vi "OAXML_Load Configuration.vi"(8 "error in (not an error)":errorcluster, 11 "config file":path) -> (0 "error out":errorcluster, 1 "DAQ Configuration out":T1 {"pregain" format="%.2f"; "IEPE" items=["On", "Off", "None"]; "coupling" items=["DC", "AC"]; "engineering units" items=["custom..."=0, "V"=1, "A"=21, "C"=30, "pC"=31, "s"=32, "-"=29, "Pa"=2, "N"=20, "g"=3, "m/s^2"=4, "m/s"=5, "m"=6, "mm/s"=12, "mm"=13, "micron/s"=14, "micron"=15, "in/s^2"=7, "in/s"=8, "in"=9, "mil/s"=10, "mil"=11, "rad/s^2"=16, "rad/s"=17, "rad"=18, "deg/s^2"=26, "deg/s"=27, "deg"=28, "RPM"=22, "cycle/s^2"=23, "Hz"=24, "cycle"=25, "strain"=19]; "sensor sensitivity (mV/EU)" format="%.2f"; "dB reference" format="%.1e"}, 2 "param out":T3, 3 "config file out":path)   [LabVIEW 2017]
uses:
  <vilib>/addons/Sound and Vibration/Order Analysis/Example Support/sub VIs/OAXML_DSA DAQ Config.ctl
  <vilib>/addons/_NISVFA/_Shared subVIs/Controls/svc_Engineering Units Text Ring.ctl
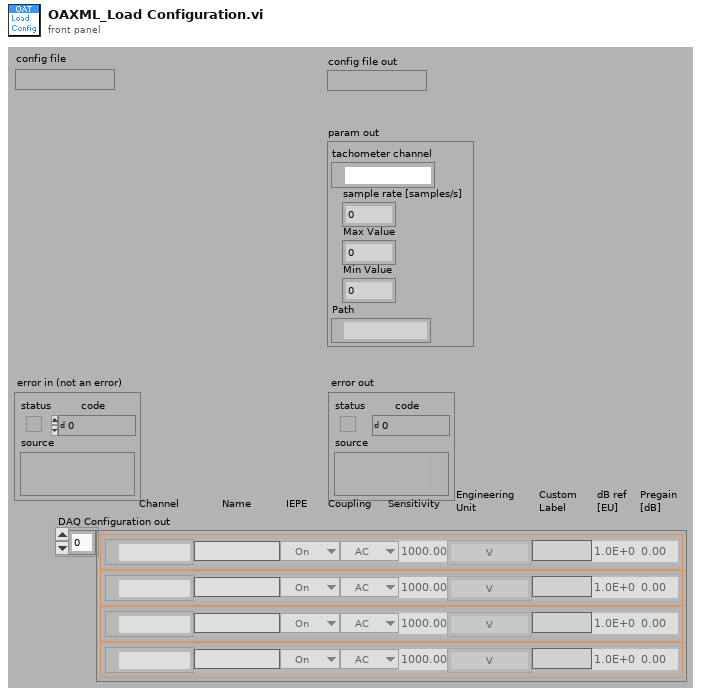
[diagram p1: front panel]
types:
  T1 = typedef "OAXML_DSA DAQ Config.ctl" = cluster{"name":string, "channel":tag, "coupling":u16, "dB reference":sgl, "sensor sensitivity (mV/EU)":dbl, "engineering units":T2, "IEPE":u16, "custom label":string, "pregain":sgl}[]
  T2 = typedef "svc_Engineering Units Text Ring.ctl" = u16
  T3 = cluster{"tachometer channel":tag, "sample rate [samples/s]":dbl, "Max Value":dbl, "Min Value":dbl, "Path":path}
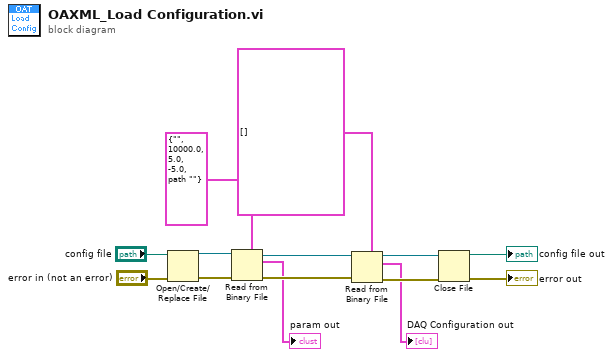
[diagram p0: block diagram]
diagram:
  n1 = Open/Create/Replace File(file path (use dialog)="config file", error in="error in (not an error)") -> (refnum out=w5:refnum<file>, error out=w11:errorcluster)  [unwired: 4 in, 1 out]
  n2 = Read from Binary File(5:T3 {"tachometer channel"="", "sample rate [samples/s]"=10000.0, "Max Value"=5.0, "Min Value"=-5.0, "Path"=path ""} ("Param in"), 8:w11, 11:w5) -> (0:w9:errorcluster, 2:→"param out":T3, 3:w10:refnum<file>)  [unwired: 3 in, 1 out]
  n3 = Read from Binary File(5:T1 [] ("DAQ Config in"), 8:w9, 11:w10) -> (0:w7:errorcluster, 2:→"DAQ Configuration out":T1, 3:w8:refnum<file>)  [unwired: 3 in, 1 out]
  n4 = Close File(refnum=w8, error in=w7) -> (path=→"config file out":path, error out=→"error out":errorcluster)
